vi "Starter Kit 2.0 Custom FPGA Main Modified.vi"(2 "PWM Right Motor":T1={"period (uSec)"=20000, "pulse width (uSec)"=1500}, 3 "PWM Left Motor":T1={"period (uSec)"=20000, "pulse width (uSec)"=1500}) -> (0 "Left cw count (pulses)":i32, 1 "Right cw count (pulses)":i32)   [LabVIEW 2013]
doc: "This VI implements the low level control of the motors and sensor for the Starter Kit 2.0 robot. The functionality of this VI is similar to the fixed FPGA personality used by the Starter Kit API."
uses:
  <vilib>/Platform/TimedLoop/XDataNode/timing_clust.ctl
  <vilib>/Platform/TimedLoop/XDataNode/nitl_modes.ctl
  <vilib>/Platform/TimedLoop/XDataNode/wakeup.ctl
  <vilib>/robotics/Utilities/Encoder Count Encoding.ctl
  <vilib>/rvi/Emulation/niFpgaSctlEmulationGetInTimedLoop.vi
  <vilib>/rvi/Emulation/niFpgaProcessEmulError.vi
  <vilib>/rvi/Emulation/niFpgaEmulationReportErrorSimple.vi
  <vilib>/rvi/Emulation/niFpgaGetClockAttributes.vi
  <vilib>/rvi/Emulation/niFpgaCriticalErrorInLSC.vi
  <vilib>/robotics/Utilities/FPGA Utilities/Count Two Phase Digital Encoder.vi
  Support VIs/Starter Kit 2.0 FPGA Globals.vi
  <vilib>/Platform/TimedLoop/XDataNode/XDataNode.xnode
  <vilib>/Platform/TimedLoop/XDataNode/XDNodeRunTimeDep.lvlib
  <vilib>/robotics/Utilities/NI_Robotics Utilities.lvlib
  <vilib>/robotics/Utilities/FPGA Utilities/NI_Robotics_FPGA Utilities.lvlib
  <instrlib>/Parallax PING)))/FPGA/NI_Robotics_Parallax PING))) (FPGA).lvlib
  <instrlib>/Hitec HS400 Series/FPGA/NI_Robotics_Hitec HS400 Series (FPGA).lvlib
panel:
  in  "hs400_0_ccw angle":fxp<+/-,32,4>
  in  "hs400_0_ccw offset":fxp<+/-,32,4>
  out "PING)))_0_timeout":bool
  out "PING)))_0_dist":fxp<+,32,8> format="%.27g"
  in  "stop":bool
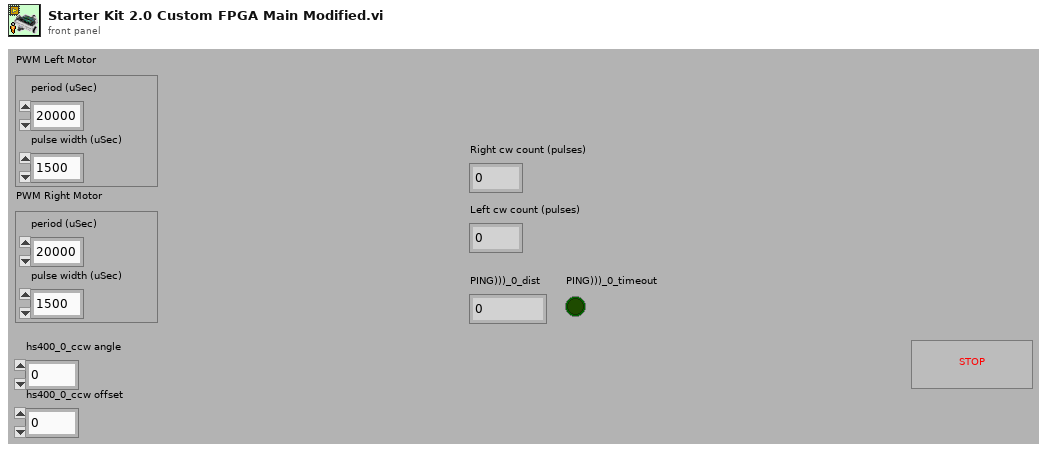
[diagram p1: front panel]
types:
  T1 = cluster{"period (uSec)":u32, "pulse width (uSec)":u32}
  T2 = typedef "XDNodeRunTimeDep.lvlib/timing_clust.ctl" = cluster{"Expected End [f-1]":u64, "Actual End [f-1]":u64, "Finished Late? [f-1]":bool, "Expected End [i-1]":u64, "Actual End [i-1]":u64, "Finished Late? [i-1]":bool, "Expected Start [i]":u64, "Actual Start [i]":u64, "Expected Start [f]":u64, "Actual Start [f]":u64, "Source Name":string, "Structure Name":string, "Period":i64, "Deadline":i64, "Offset":i64, "Start":i64, "Priority":i32, "Timeout":i32, "Mode":T3, "Wakeup Reason":T4, "Error":errorcluster, "Source Type":string, "Secondary Source Type":string, "Global End Time":u64, "Global Start Time":u64, "Frame Duration":u64, "Iteration Duration":u64, "Assigned CPU":i32, "I/O Scan Engine Mode":u32}
  T3 = typedef "XDNodeRunTimeDep.lvlib/nitl_modes.ctl" = enum32{"No Change", "Process missed periods, maintain original phase", "Discard missed periods, maintain original phase", "Process missed periods, ignore original phase", "Discard missed periods, ignore original phase"}
  T4 = typedef "XDNodeRunTimeDep.lvlib/wakeup.ctl" = enum32{"Normal", "Aborted", "Asynchronous wakeup", "Timing source error", "Timed loop error", "Timeout"}
  T5 = typedef "NI_Robotics Utilities.lvlib/Encoder Count Encoding.ctl" = enum16{"X1", "X2", "X4"}
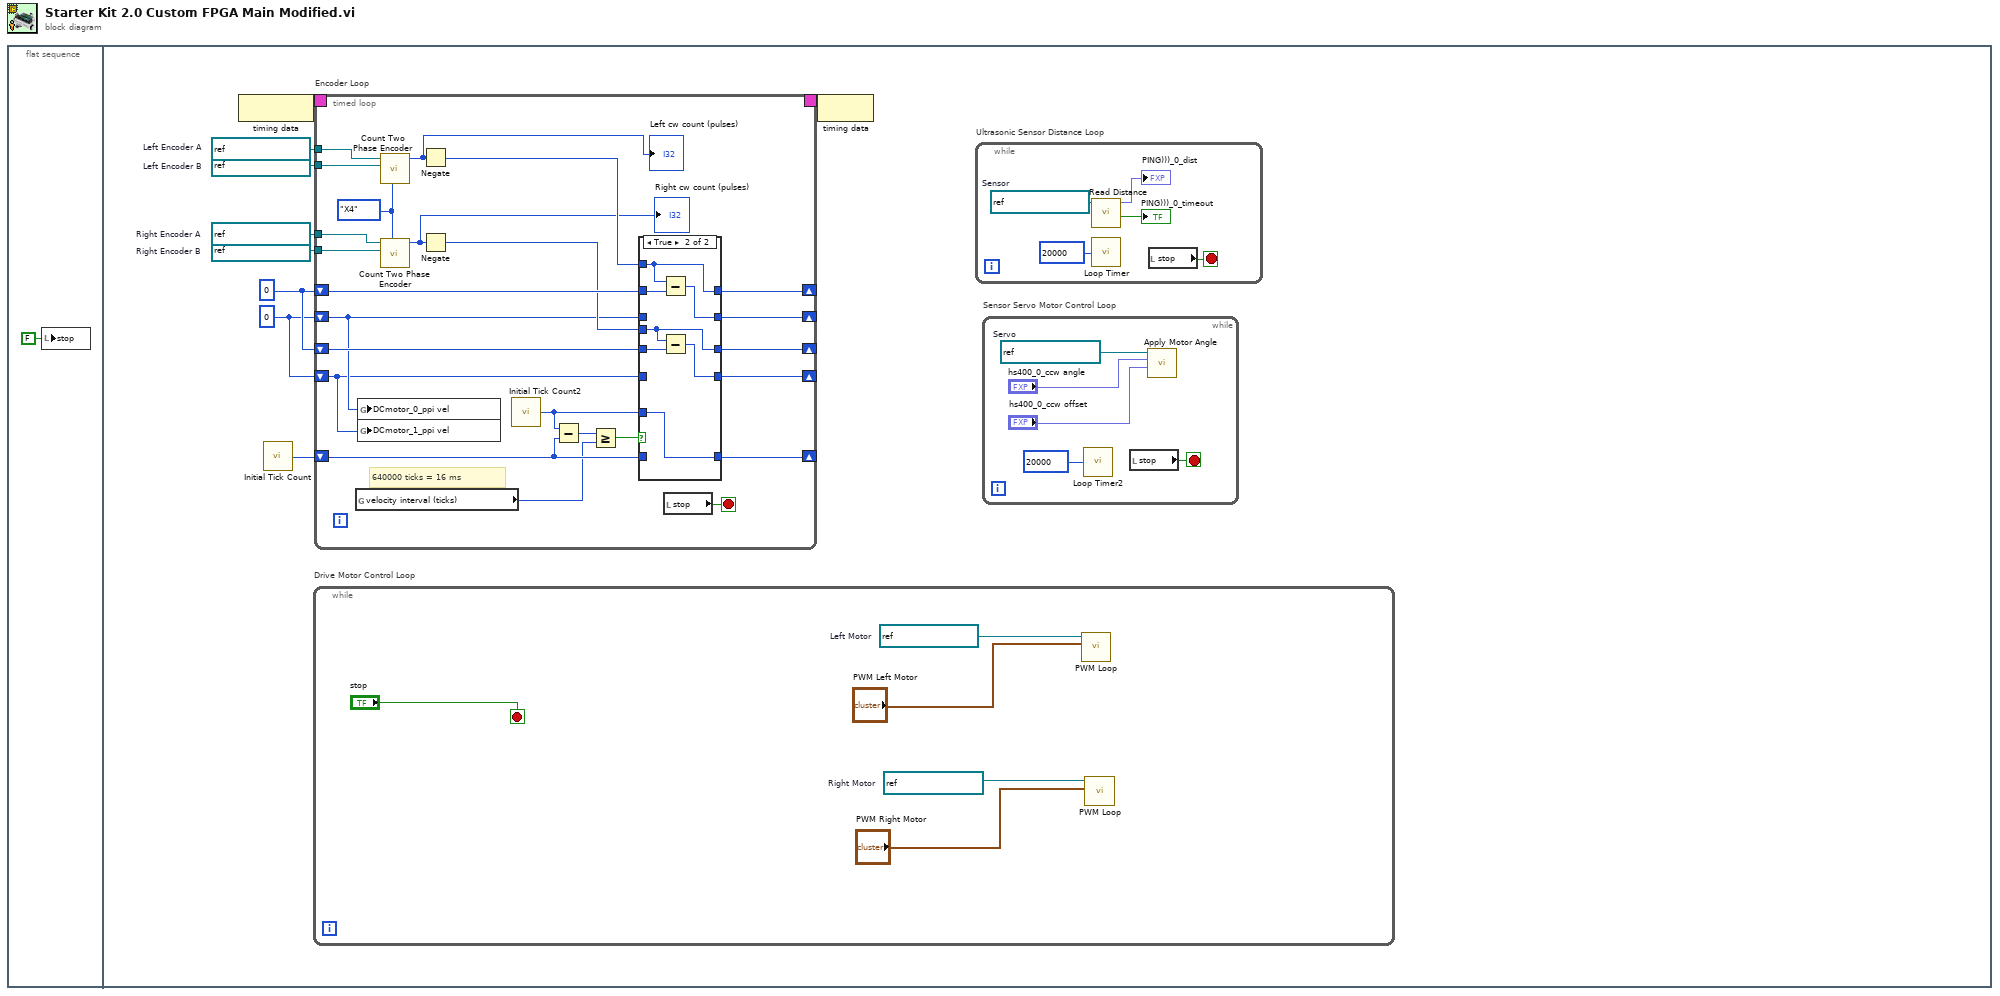
[diagram p0: block diagram]
diagram:
  n1 = flat-sequence {
    frame #0 {
      n2 = local write "stop"(FALSE ("stop")) -> ()
    }
    frame #1 {
      w2 = refnum<k21> "Port0/DIO3"  # Right Encoder B
      w3 = refnum<k21> "Port0/DIO2"  # Right Encoder A
      w4 = refnum<k21> "Port0/DIO1"  # Left Encoder B
      w5 = refnum<k21> "Port0/DIO0"  # Left Encoder A
      w6 = 0
      w7 = 0 ("Reset Position Value")
      n3 = node-c288() -> (w10:T2)
      n4 = call "Initial Tick Count"() -> ("Tick Count(Ticks)"=w8:u32)
      n5 = while "Drive Motor Control Loop" {
        stop <- "stop" stop-if-true
        w22 = refnum<k21> "Port0/DIO5"  # Right Motor
        w24 = refnum<k21> "Port0/DIO4"  # Left Motor
        n6 = call "PWM Loop.vi"("PWM"="PWM Left Motor", "FPGA I/O"=w24) -> ()  [unwired: 10 in]
        n7 = call "PWM Loop.vi"("PWM"="PWM Right Motor", "FPGA I/O"=w22) -> ()  [unwired: 10 in]
      }
      n8 = timed-loop "Encoder Loop" {
        timing: w10 -> [_]
        timing-out: [_] -> w9
        shift-right: [w42] -> _
        shift-left: w8 -> [w47]
        shift-right: [w43] -> _
        shift-left: w7 -> [w45]
        shift-right: [w44] -> _
        shift-left: w6 -> [w30]
        shift-right: [w40] -> _
        shift-left: w7 -> [w41]
        shift-right: [w39] -> _
        shift-left: w6 -> [w29]
        tunnel: w5 -> [w35]
        tunnel: w4 -> [w34]
        tunnel: w3 -> [w33]
        tunnel: w2 -> [w32]
        stop <- w36 stop-if-true
        w31 = Encoder_Count_Encoding."X4" ("count multiplier (X1)")
        # "640000 ticks = 16 ms"
        n9 = global read "Starter Kit 2.0 FPGA Globals.vi" "velocity interval (ticks)"() -> (w28:u32)
        n10 = global write "Starter Kit 2.0 FPGA Globals.vi" "DCmotor_0_ppi vel"(w30) -> ()
        n11 = global write "Starter Kit 2.0 FPGA Globals.vi" "DCmotor_1_ppi vel"(w29) -> ()
        n12 = call-poly <vilib>:"Count Two Phase Encoder.vi"("count encoding (X1)"=w31, "phase B FPGA digital input"=w34, "phase A FPGA digital input"=w35) -> ("new count"=w27:i32)  [unwired: 7 in, 1 out]
        "Left cw count (pulses)" <- w27
        n13 = call-poly <vilib>:"Count Two Phase Encoder.vi"("count encoding (X1)"=w31, "phase B FPGA digital input"=w32, "phase A FPGA digital input"=w33) -> ("new count"=w26:i32)  [unwired: 7 in, 1 out]
        "Right cw count (pulses)" <- w26
        n14 = Negate(x=w27) -> (-x=w38:i32)
        n15 = Negate(x=w26) -> (-x=w37:i32)
        n16 = call "Initial Tick Count2"() -> ("Tick Count(Ticks)"=w46:u32)
        n17 = Subtract(x=w46, y=w47) -> (x-y=w49:u32)
        n18 = Greater Or Equal?(x=w49, y=w28) -> (x >= y?=w48:bool)
        n19 = case shown="True" w48 {
          tunnel: w46 -> [_ w60]
          tunnel: w47 -> [w54 _]
          tunnel: [w54 w60] -> w42
          tunnel: w45 -> [w53 w61]
          tunnel: [w53 w59] -> w43
          tunnel: w38 -> [_ w59]
          tunnel: [w52 w58] -> w44
          tunnel: w30 -> [w52 _]
          tunnel: w41 -> [w51 w57]
          tunnel: w29 -> [w50 _]
          tunnel: [w51 w56] -> w40
          tunnel: [w50 w55] -> w39
          tunnel: w37 -> [_ w56]
          frame False {
          }
          frame True {
            n20 = Subtract(x=w59, y=w61) -> (x-y=w58:i32)
            n21 = Subtract(x=w56, y=w57) -> (x-y=w55:i32)
          }
        }
        n22 = local read "stop"() -> (w36:bool)
      }
      n23 = node-c288(w9) -> ()
      n24 = while "Ultrasonic Sensor Distance Loop" {
        stop <- w19 stop-if-true
        w16 = refnum<k21> "Port0/DIO6"  # Sensor
        n25 = call <instrlib>:"Read Distance.vi"("trigger/echo line"=w16) -> ("timed out?"=→"PING)))_0_timeout":bool, "distance (m)"=→"PING)))_0_dist":fxp<+,32,8>)  [unwired: 9 in]
        n26 = call "Loop Timer"("Count(uSec)"=u32 20000 ("sensor period (15000 us)")) -> ()  [unwired: 1 out]
        n27 = local read "stop"() -> (w19:bool)
      }
      n28 = while "Sensor Servo Motor Control Loop" {
        stop <- w15 stop-if-true
        w14 = refnum<k21> "Port0/DIO7"  # Servo
        n29 = call "Loop Timer2"("Count(uSec)"=u32 20000) -> ()  [unwired: 1 out]
        n30 = local read "stop"() -> (w15:bool)
        n31 = call <instrlib>:"Apply Motor Angle.vi"("ccw angle offset (rad)"="hs400_0_ccw offset", "ccw angle (rad)"="hs400_0_ccw angle", "digital output line"=w14) -> ()  [unwired: 9 in]
      }
    }
  }
